vi "HoppingStep.vi"() -> ()   [LabVIEW 2014]
uses:
  <vilib>/Platform/TimedLoop/XDataNode/timing_clust.ctl
  <vilib>/Platform/TimedLoop/XDataNode/nitl_modes.ctl
  <vilib>/Platform/TimedLoop/XDataNode/wakeup.ctl
  <vilib>/rvi/Emulation/niFpgaGetClockAttributes.vi
  <vilib>/rvi/Emulation/niFpgaSctlEmulationGetInTimedLoop.vi
  <vilib>/rvi/Emulation/niFpgaEmulationReportErrorSimple.vi
  <vilib>/rvi/eio/common/nirviEmuTemplateMethod_errors.vi
  <vilib>/rvi/Emulation/niFpgaCriticalErrorInLSC.vi
  <vilib>/rvi/interface/RandomDataEmulation/niFpgaRandomDataHandleErrors.vi
  <vilib>/eio/EIONode/EIONode.xnode
  <vilib>/Platform/TimedLoop/XDataNode/XDataNode.xnode
  <vilib>/rvi/DataTransferAndStorage/Container/XNode/niFpgaContainer.xnode
  <vilib>/rvi/interface/RandomDataEmulation/nirviRandomDataFpgaReadWriteTemplate.vi
  <vilib>/Platform/TimedLoop/XDataNode/XDNodeRunTimeDep.lvlib
panel:
  in  "stop":bool
  in  "XStepIndex":i16
  in  "XNum":i16
  in  "XOffset":i16
  in  "ZOffset":i16
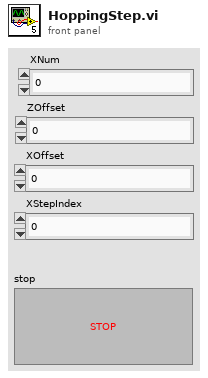
[diagram p1: front panel]
types:
  T1 = typedef "XDNodeRunTimeDep.lvlib/timing_clust.ctl" = cluster{"Expected End [f-1]":u64, "Actual End [f-1]":u64, "Finished Late? [f-1]":bool, "Expected End [i-1]":u64, "Actual End [i-1]":u64, "Finished Late? [i-1]":bool, "Expected Start [i]":u64, "Actual Start [i]":u64, "Expected Start [f]":u64, "Actual Start [f]":u64, "Source Name":string, "Structure Name":string, "Period":i64, "Deadline":i64, "Offset":i64, "Start":i64, "Priority":i32, "Timeout":i32, "Mode":T2, "Wakeup Reason":T3, "Error":errorcluster, "Source Type":string, "Secondary Source Type":string, "Global End Time":u64, "Global Start Time":u64, "Frame Duration":u64, "Iteration Duration":u64, "Assigned CPU":i32, "I/O Scan Engine Mode":u32}
  T2 = typedef "XDNodeRunTimeDep.lvlib/nitl_modes.ctl" = enum32{"No Change", "Process missed periods, maintain original phase", "Discard missed periods, maintain original phase", "Process missed periods, ignore original phase", "Discard missed periods, ignore original phase"}
  T3 = typedef "XDNodeRunTimeDep.lvlib/wakeup.ctl" = enum32{"Normal", "Aborted", "Asynchronous wakeup", "Timing source error", "Timed loop error", "Timeout"}
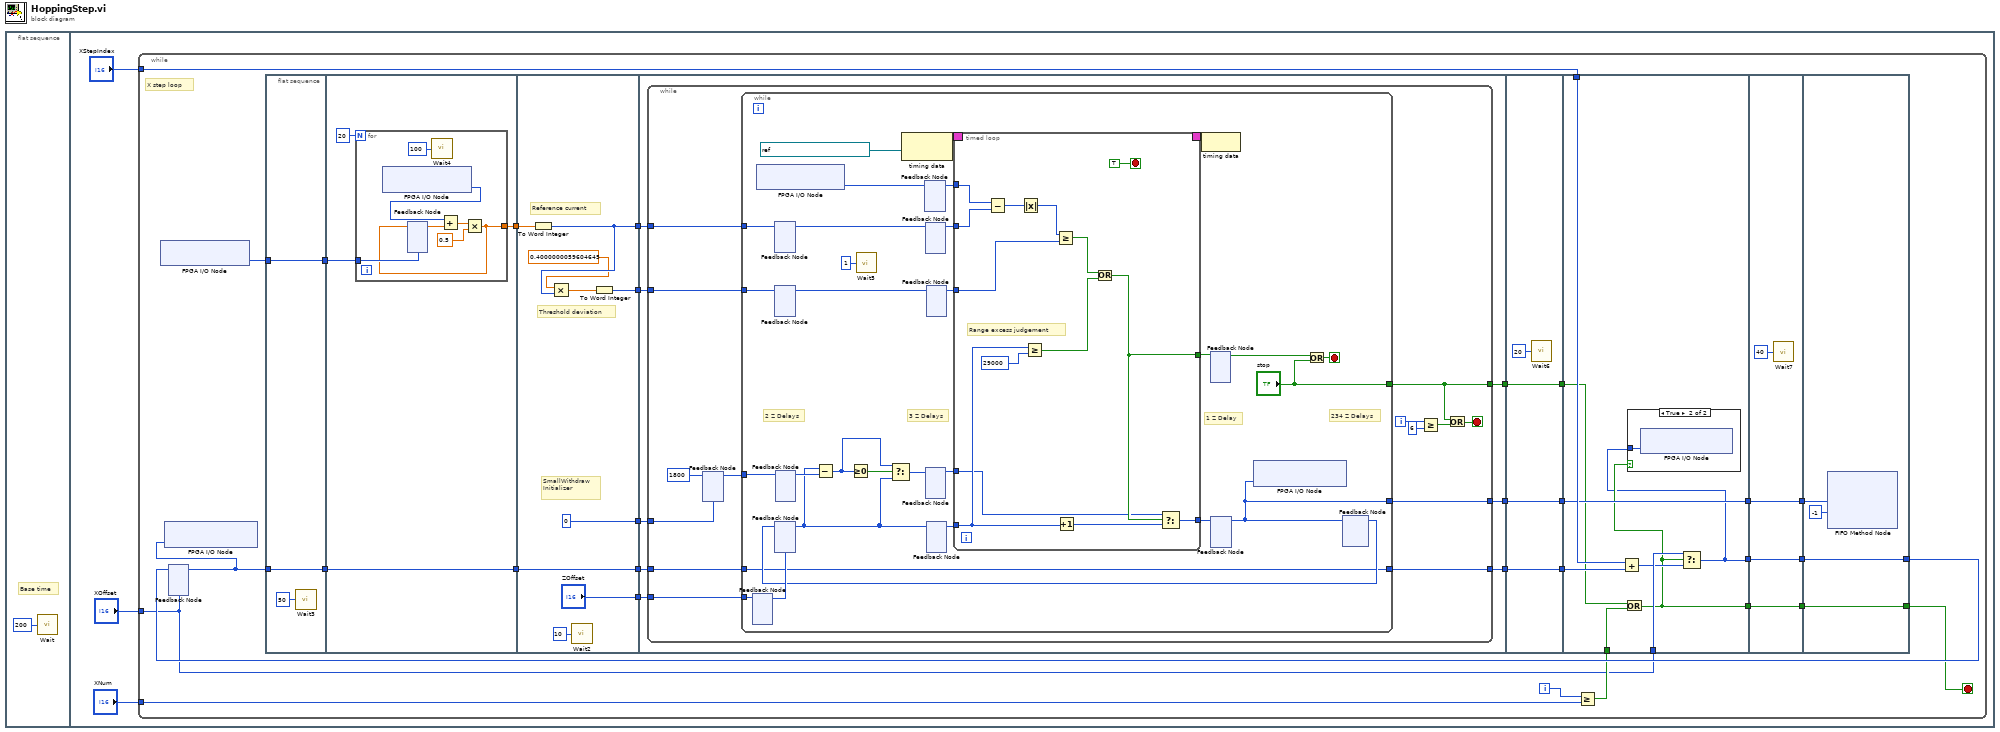
[diagram p0: block diagram]
diagram:
  n1 = flat-sequence {
    frame #0 {
      # "Base time"
      n2 = call "Wait"("Count(uSec)"=u32 200) -> ()  [unwired: 1 out]
    }
    frame #1 {
      n3 = while {
        tunnel: "XOffset" -> [w8]
        tunnel: "XNum" -> [w17]
        tunnel: "XStepIndex" -> [w25]
        i -> [w16]
        stop <- w5 stop-if-true
        # "X step loop"
        n4 = xnode "FPGA I/O Node"() -> ("Connector0/AI1"=w18:i16)  [unwired: 1 in, 1 out]
        n5 = feedback #1(w8) -> (w20:i16)
        n6 = xnode "FPGA I/O Node"("Connector0/AO2"=w20) -> ()  [unwired: 1 in, 1 out]
        n7 = feedback-in #1(w19) -> ()
        n8 = flat-sequence {
          tunnel: [w37] -> w32
          tunnel: [w35] -> w30
          tunnel: w20 -> [w37]
          tunnel: w18 -> [w35]
          tunnel: w32 -> [w41]
          tunnel: [w41] -> w33
          tunnel: w30 -> [w40]
          tunnel: [w38] -> w29
          tunnel: ["ZOffset"] -> w34
          tunnel: w33 -> [w55]
          tunnel: [w55] -> w31
          tunnel: w29 -> [w54]
          tunnel: [w53] -> w28
          tunnel: [w50] -> w27
          tunnel: [i16 0] -> w26
          tunnel: w26 -> [w61]
          tunnel: w27 -> [w62]
          tunnel: w28 -> [w63]
          tunnel: w31 -> [w65]
          tunnel: w34 -> [w64]
          tunnel: [w60] -> w23
          tunnel: [w59] -> w21
          tunnel: [w58] -> w10
          tunnel: [w132] -> w24
          tunnel: w23 -> [w132]
          tunnel: [w131] -> w22
          tunnel: w21 -> [w131]
          tunnel: [w130] -> w11
          tunnel: w10 -> [w130]
          tunnel: w25 -> [w141]
          tunnel: w24 -> [w140]
          tunnel: w22 -> [w142]
          tunnel: [w134] -> w15
          tunnel: [w140] -> w14
          tunnel: w11 -> [w139]
          tunnel: w9 -> [w138]
          tunnel: w8 -> [w137]
          tunnel: [w135] -> w6
          tunnel: w15 -> [w147]
          tunnel: w14 -> [w145]
          tunnel: [w147] -> w13
          tunnel: [w145] -> w12
          tunnel: [w144] -> w7
          tunnel: w6 -> [w144]
          tunnel: [w151] -> w19
          tunnel: w13 -> [w151]
          tunnel: w12 -> [w150]
          tunnel: [w148] -> w5
          tunnel: w7 -> [w148]
          frame #0 {
            n9 = call "Wait3"("Count(uSec)"=u32 50) -> ()  [unwired: 1 out]
          }
          frame #1 {
            n10 = for {
              N: 20 -> [_]
              tunnel: w40 -> [w47]
              tunnel: [w42] -> w38
              n11 = xnode "FPGA I/O Node"() -> ("Connector0/AI1"=w45:i16)  [unwired: 1 in, 1 out]
              n12 = feedback #2(w47) -> (w46:sgl)
              n13 = call "Wait4"("Count(uSec)"=u32 100) -> ()  [unwired: 1 out]
              n14 = Add(x=w45, y=w46) -> (x+y=w44:sgl)
              n15 = Multiply(x=w44, y=sgl 0.5) -> (x*y=w42:sgl)
              n16 = feedback-in #2(w42) -> ()
            }
          }
          frame #2 {
            # "SmallWithdraw\nInitializer"
            # "Threshold deviation"
            # "Reference current"
            n17 = To Word Integer(number=w54) -> (16bit integer=w53:i16)
            n18 = Multiply(x=sgl 0.4, y=w53) -> (x*y=w51:sgl)
            n19 = call "Wait2"("Count(uSec)"=u32 10) -> ()  [unwired: 1 out]
            n20 = To Word Integer(number=w51) -> (16bit integer=w50:i16)
          }
          frame #3 {
            n21 = while {
              tunnel: w65 -> [w79]
              tunnel: w64 -> [w78]
              tunnel: w63 -> [w77]
              tunnel: w62 -> [w76]
              tunnel: w61 -> [w74]
              tunnel: [w70] -> w60
              tunnel: [w69] -> w59
              tunnel: [w66] -> w58
              i -> [w72]
              stop <- w68 stop-if-true
              n22 = feedback #3(w74) -> (w75:i16)
              n23 = feedback-in #3(i16 1800) -> ()
              n24 = while {
                tunnel: w79 -> [w92]
                tunnel: w78 -> [w97]
                tunnel: w77 -> [w108]
                tunnel: w76 -> [w109]
                tunnel: w75 -> [w98]
                tunnel: [w92] -> w69
                tunnel: [w91] -> w70
                tunnel: ["stop"] -> w66
                stop <- w82 stop-if-true
                # "234 Z Delays"
                # "1 Z Delay"
                # "3 Z Delays"
                # "2 Z Delays"
                n25 = feedback #4() -> (w96:i16)  [unwired: 1 in]
                n26 = feedback-in #4(w97) -> ()
                n27 = xnode "FPGA I/O Node"() -> ("Connector0/AI1"=w90:i16)  [unwired: 1 in, 1 out]
                n28 = feedback #5() -> (w103:i16)  [unwired: 1 in]
                n29 = feedback-in #5(w108) -> ()
                n30 = feedback #6() -> (w101:i16)  [unwired: 1 in]
                n31 = feedback-in #6(w109) -> ()
                n32 = feedback #7(w96) -> (w86:i16)
                n33 = feedback #8() -> (w87:i16)  [unwired: 1 in]
                n34 = feedback-in #8(w98) -> ()
                n35 = Subtract(x=w86, y=w87) -> (x-y=w83:i16)
                n36 = Greater Or Equal To 0?(x=w83) -> (x >= 0?=w88:bool)
                n37 = call "Wait5"("Count(uSec)"=u32 1) -> ()  [unwired: 1 out]
                n38 = Select(t=w83, s=w88, f=w86) -> (s? t:f=w85:i16)
                n39 = node-c288(refnum<k21> "40 MHz Onboard Clock" ("Source Name")) -> (w107:T1)
                n40 = feedback #9() -> (w89:i16)  [unwired: 1 in]
                n41 = feedback-in #9(w90) -> ()
                n42 = feedback #10() -> (w102:i16)  [unwired: 1 in]
                n43 = feedback-in #10(w103) -> ()
                n44 = feedback #11() -> (w84:i16)  [unwired: 1 in]
                n45 = feedback-in #11(w85) -> ()
                n46 = feedback #12() -> (w100:i16)  [unwired: 1 in]
                n47 = feedback-in #12(w101) -> ()
                n48 = feedback #13() -> (w99:i16)  [unwired: 1 in]
                n49 = feedback-in #13(w86) -> ()
                n50 = timed-loop {
                  timing: w107 -> [_]
                  timing-out: [_] -> w106
                  tunnel: w102 -> [w120]
                  tunnel: w100 -> [w117]
                  tunnel: w89 -> [w121]
                  tunnel: w99 -> [w114]
                  tunnel: [w112] -> w95
                  tunnel: [w111] -> w94
                  tunnel: w84 -> [w110]
                  stop <- TRUE stop-if-true
                  # "Range excess judgement"
                  n51 = Subtract(x=w121, y=w120) -> (x-y=w119:i16)
                  n52 = Absolute Value(x=w119) -> (abs(x)=w118:i16)
                  n53 = Greater Or Equal?(x=w114, y=i16 29000) -> (x >= y?=w115:bool)
                  n54 = Greater Or Equal?(x=w118, y=w117) -> (x >= y?=w116:bool)
                  n55 = Increment(x=w114) -> (x+1=w113:i16)
                  n56 = Or(x=w116, y=w115) -> (x .or. y?=w111:bool)
                  n57 = Select(t=w110, s=w111, f=w113) -> (s? t:f=w112:i16)
                }
                n58 = node-c288(w106) -> ()
                n59 = feedback #14() -> (w81:bool)  [unwired: 1 in]
                n60 = feedback-in #14(w94) -> ()
                n61 = feedback #15() -> (w91:i16)  [unwired: 1 in]
                n62 = feedback-in #15(w95) -> ()
                n63 = xnode "FPGA I/O Node"("Connector0/AO0"=w91) -> ()  [unwired: 1 in, 1 out]
                n64 = Or(x=w81, y="stop") -> (x .or. y?=w82:bool)
                n65 = feedback #16() -> (w93:i16)  [unwired: 1 in]
                n66 = feedback-in #7(w93) -> ()
                n67 = feedback-in #16(w91) -> ()
              }
              n68 = Greater Or Equal?(x=w72, y=6) -> (x >= y?=w67:bool)
              n69 = Or(x=w66, y=w67) -> (x .or. y?=w68:bool)
            }
          }
          frame #4 {
            n70 = call "Wait6"("Count(uSec)"=u32 20) -> ()  [unwired: 1 out]
          }
          frame #5 {
            n71 = Add(x=w141, y=w142) -> (x+y=w136:i16)
            n72 = Or(x=w139, y=w138) -> (x .or. y?=w135:bool)
            n73 = Select(t=w137, s=w135, f=w136) -> (s? t:f=w134:i16)
            n74 = case shown="True" w135 {
              tunnel: w134 -> [_ w143]
              frame False {
              }
              frame True {
                n75 = xnode "FPGA I/O Node"("Connector0/AO2"=w143) -> ()  [unwired: 1 in, 1 out]
              }
            }
          }
          frame #6 {
            n76 = call "Wait7"("Count(uSec)"=u32 40) -> ()  [unwired: 1 out]
          }
          frame #7 {
            n77 = xnode ("FIFO Method Node")("Element"=w150, "Timeout"=-1) -> ()  [unwired: 1 in, 2 out]
          }
        }
        n78 = Greater Or Equal?(x=w16, y=w17) -> (x >= y?=w9:bool)
      }
    }
  }
